vi "(SubVI)Voltage Range to Byte Value.vi"(11 "Voltage Range":dbl format="%#_13g") -> (2 "Valid":bool, 3 "Byte Value":u8)   [LabVIEW 2020]
uses:
  Variables/(Var)System Variables.vi
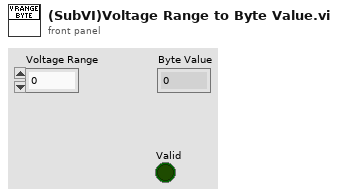
[diagram p1: front panel]
types:
  T1 = typedef "Haptic IC.lvclass/(Ctrl)IC Type.ctl" = enum8{"DW7800", "DW7912", "DW7914"}
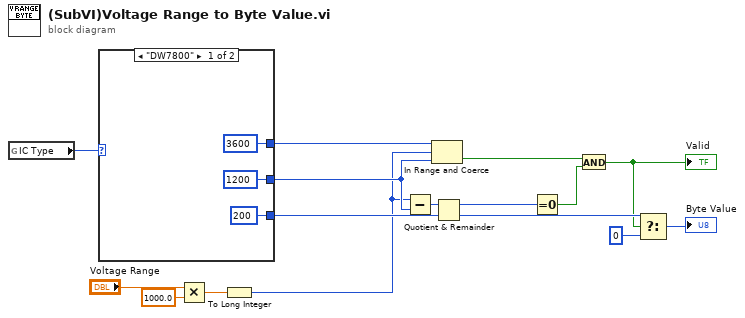
[diagram p0: block diagram]
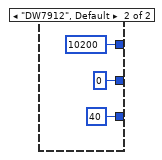
[diagram p2: hidden frame]
diagram:
  n1 = global read "(Var)System Variables.vi" "IC Type"() -> (w16:T1)
  n2 = case shown="\"DW7800\"" w16 {
    tunnel: [3600 ("Max") 10200 ("Max")] -> w15
    tunnel: [1200 ("Min") 0 ("Min")] -> w9
    tunnel: [200 ("Increment") 40 ("Increment")] -> w12
    frame "DW7800" {
    }
    frame "DW7912", Default {
    }
  }
  n3 = Multiply(x="Voltage Range", y=1000.0) -> (x*y=w10:dbl)
  n4 = To Long Integer(number=w10) -> (32bit integer=w8:i32)
  n5 = Subtract(x=w8, y=w9) -> (x-y=w11:i32)
  n6 = In Range and Coerce(upper limit=w15, x=w8, lower limit=w9) -> (In Range?=w7:bool)  [unwired: 1 out]
  n7 = Quotient & Remainder(x=w11, y=w12) -> (x-y*floor(x/y)=w5:i32, floor(x/y)=w4:i32)
  n8 = Equal To 0?(x=w5) -> (x = 0?=w6:bool)
  n9 = And(x=w7, y=w6) -> (x .and. y?=w3:bool)
  "Valid" <- w3
  n10 = Select(t=w4, s=w3, f=0) -> (s? t:f=→"Byte Value":i32)
